vi "Points to Oval2.vi"(8 "Size":dbl, 9 "Y":dbl[](array[numeric]), 10 "X":dbl[](array[numeric]), 11 "Image In":T1) -> (3 "Image Out":T1(plugin-control))   [LabVIEW 2017]
uses:
  <vilib>/vision/Image Controls.llb/IMAQ Image.ctl
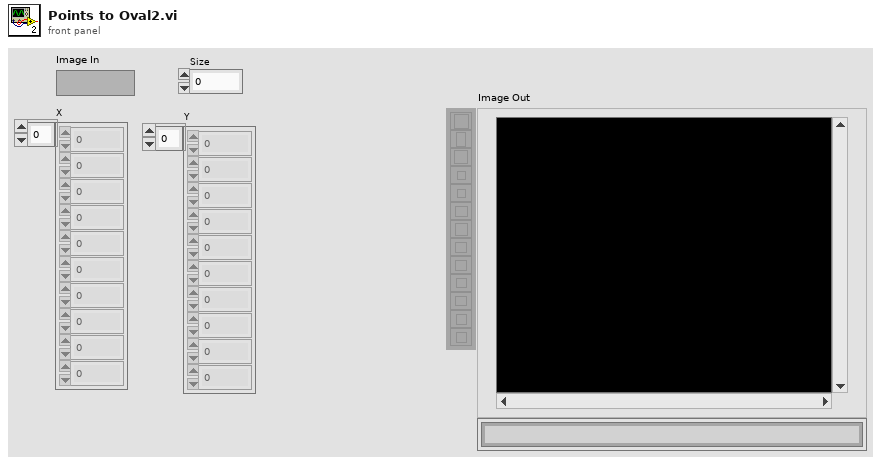
[diagram p1: front panel]
types:
  T1 = typedef "IMAQ Image.ctl" = refnum<image>
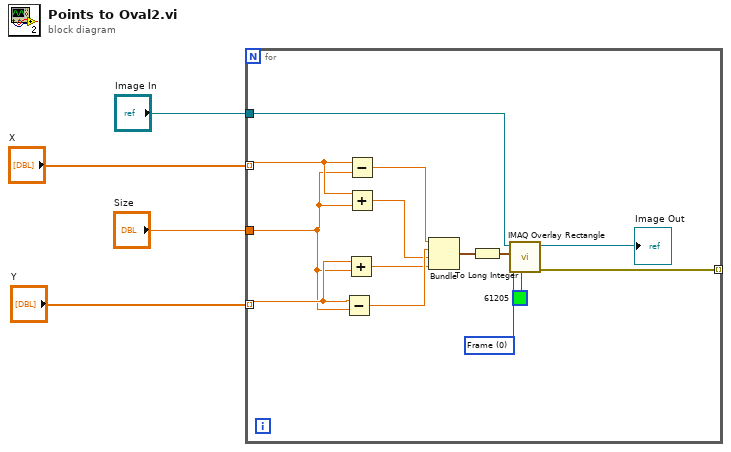
[diagram p0: block diagram]
diagram:
  n1 = for {
    tunnel: "X" -> [w16] mode=indexing
    tunnel: "Y" -> [w14] mode=indexing
    tunnel: "Size" -> [w12]
    tunnel: "Image In" -> [w10]
    tunnel: [w5] -> _ mode=indexing
    w8 = u32 0 items=["Frame", "Fill"] ("Drawing Mode (Frame)")
    n2 = Subtract(x=w14, y=w12) -> (x-y=w17:dbl)
    n3 = Add(x=w14, y=w12) -> (x+y=w13:dbl)
    n4 = Subtract(x=w16, y=w12) -> (x-y=w18:dbl)
    n5 = Add(x=w16, y=w12) -> (x+y=w15:dbl)
    n6 = Bundle(w18, w17, w15, w13) -> (w7:cluster{dbl, dbl, dbl, dbl})  [unwired: 1 in]
    n7 = To Long Integer(number=w7) -> (32bit integer=w6:cluster{i32, i32, i32, i32})
    n8 = call "IMAQ Overlay Rectangle"("Color"=u32 61205, "Drawing Mode (Frame)"=w8, "Rectangle"=w6, "Image"=w10) -> ("error out"=w5:errorcluster, "Image Out"=→"Image Out":T1)  [unwired: 6 in]
  }
